vi "Initialize.vi"(8 "error in (no error)":errorcluster, 11 "Stage in":refnum<class "Stage.lvclass">) -> (0 "error out":errorcluster, 3 "Stage out":refnum<class "Stage.lvclass">)   [LabVIEW 2020]
uses:
  Stage.lvclass
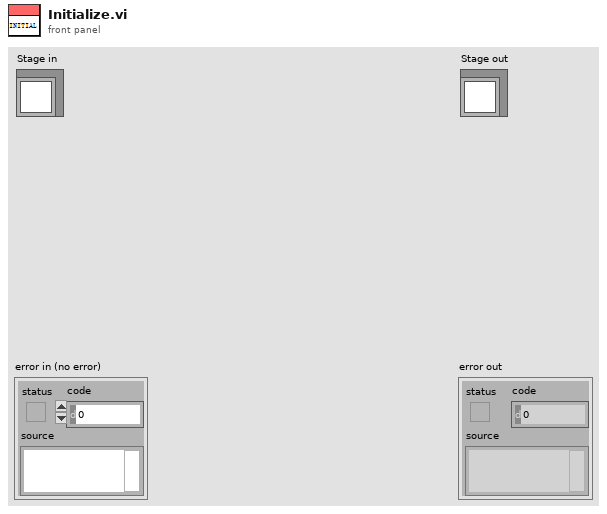
[diagram p1: front panel]
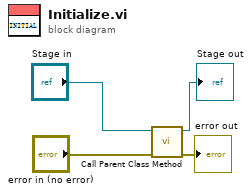
[diagram p0: block diagram]
diagram:
  n1 = call-parent "Call Parent Class Method"("error in (no error)"="error in (no error)", "Device in"="Stage in") -> ("error out"=→"error out":errorcluster, "Device out"=→"Stage out":refnum<class "Stage.lvclass">)  [unwired: 8 in]
